vi "Broadcasting.vi"(8 "error in (no error)":errorcluster, 10 "Boradcast Data":variant, 11 "Observer in":refnum<class "Observer.lvclass">) -> (0 "error out":errorcluster, 3 "Observer out":refnum<class "Observer.lvclass">)   [LabVIEW 2019, in "Observer.lvclass"]
uses:
  Observer.lvclass
  Observer.lvclass/Observer.ctl
  Subscriber/Subscriber.lvclass
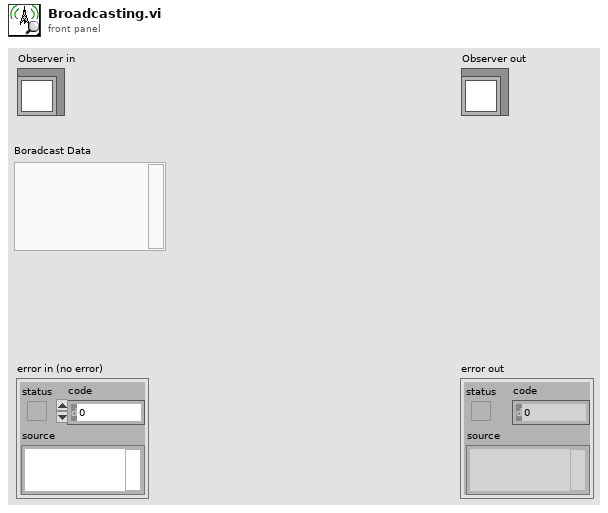
[diagram p1: front panel]
types:
  T1 = typedef "Subcribe Set.ctl" = set{refnum<class "Subscriber.lvclass">}
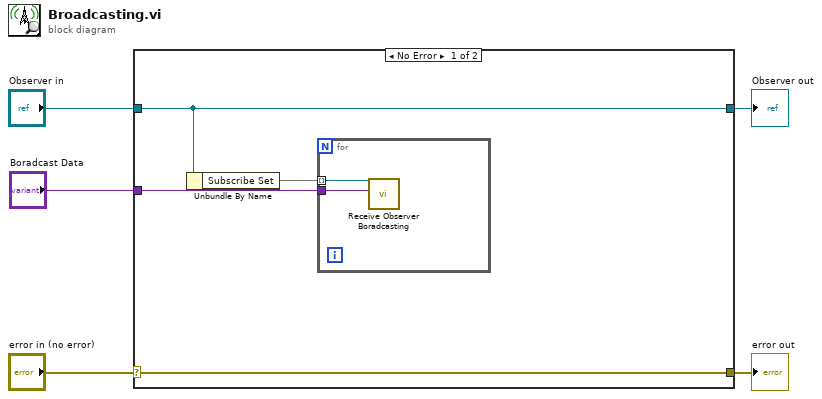
[diagram p0: block diagram]
diagram:
  n1 = case shown="No Error" "error in (no error)" {
    selector: "error in (no error)" -> [w9 w13]
    tunnel: [w9 w13] -> w4
    tunnel: [w8 w12] -> w2
    tunnel: "Observer in" -> [w8 w12]
    tunnel: "Boradcast Data" -> [w6 _]
    frame No Error {
      n2 = Unbundle By Name(w8) -> ("Subscribe Set"=w7:T1)
      n3 = for {
        tunnel: w7 -> [w11] mode=indexing
        tunnel: w6 -> [w10]
        n4 = call-dynamic "Receive Observer Boradcasting.vi"("Boradcasting Data"=w10, "Subscriber in"=w11) -> ()  [unwired: 8 in, 2 out]
      }
    }
    frame Error {
    }
  }
  "error out" <- w4
  "Observer out" <- w2
